vi "rql_Generate Error.vi"(4 "Show in Debugger?":bool=TRUE, 6 "Message Priority":T1=enum."Normal", 8 "error in":errorcluster, 10 "Data in":T2, 11 "Worker A in":refnum<class "Worker A.lvclass">) -> (0 "error out":errorcluster, 3 "dup Worker A out":refnum<class "Worker A.lvclass">)   [LabVIEW 2017, in "Worker A.lvclass"]
doc: "This VI sends a <b>Local API Request</b> message to an MHL case of the Worker that owns this VI.\n---\nCreate a random error at a rate of 1 second"
uses:
  Worker A.lvclass
  C:/Program Files (x86)/National Instruments/LabVIEW 2017/vi.lib/addons/_Workers/Library/Classes/Worker/Worker.lvclass
  rql_Generate Error.ctl
  <vilib>/addons/_Workers/Library/Classes/Message/Priority.ctl
  <vilib>/addons/_Workers/Library/Case Label.ctl
  <vilib>/addons/_Workers/Library/Classes/Message Queue/Message Queue.lvclass
  <vilib>/addons/_Workers/Library/Workers.lvlib
  <vilib>/addons/_Workers/Library/Classes/Message/Message.lvclass
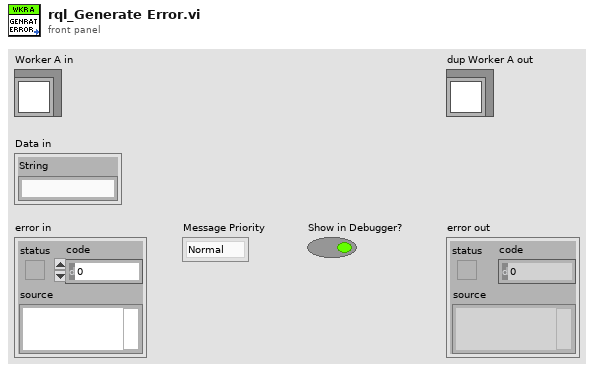
[diagram p1: front panel]
types:
  T1 = typedef "Workers.lvlib/Message.lvclass/Priority.ctl" = enum16{"Low", "Normal", "High"}
  T2 = typedef "Worker A.lvclass/rql_Generate Error.ctl" = cluster{"String":string}
  T3 = typedef "Workers.lvlib/Case Label.ctl" = string
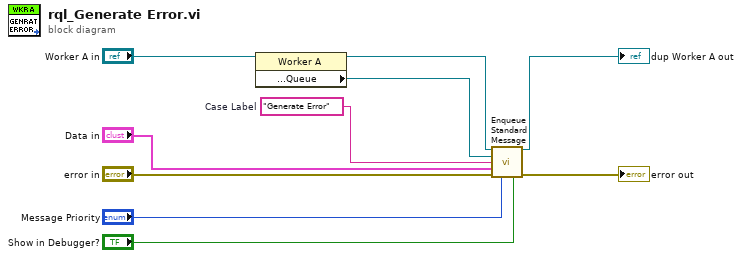
[diagram p0: block diagram]
diagram:
  w1 = T3 "Generate Error"  # Case Label
  n1 = property class="Worker A"(reference="Worker A in") -> (reference out=w3:refnum<class "Worker A.lvclass">, "Accessors:Read:Public API:Queue"=w2:refnum<class "Message Queue.lvclass">)  [unwired: 1 in, 1 out]
  n2 = call-dynamic "Enqueue Standard Message.vi"("Worker"=w3, "Message Queue"=w2, "Case Label"=w1, "Data"="Data in", "error in (no error)"="error in", "Priority (Normal)"="Message Priority", "Send Message to Debugger? (T)"="Show in Debugger?") -> ("dup Worker out"=→"dup Worker A out":refnum<class "Worker A.lvclass">, "error out"=→"error out":errorcluster)  [unwired: 7 in]
